vi "YawFromStart.vi"(11 "navX Device":T1 {"Interface"."Update Rate (4Hz-60Hz)" min=4 max=60 step=1}) -> (3 "Yaw":dbl)   [LabVIEW 2015]
uses:
  NavX/navX Library v2/TypeDefs/Z900_navX_DeviceTypeDef.ctl
  NavX/navX Library v2/TypeDefs/Z900_navX_ProtocolTypeDef.ctl
  NavX/navX Library v2/TypeDefs/Z900_navX_NotifyPacketTypeDef.ctl
  NavX/navX Library v2/TypeDefs/Z900_navX_ActionTypeDef.ctl
  Framework/Robot Global Data.vi
  NavX/navX Library v2/navX Library v2.lvlib
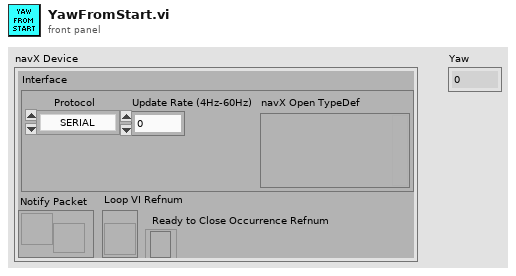
[diagram p1: front panel]
types:
  T1 = typedef "navX Library v2.lvlib/Z900_navX_DeviceTypeDef.ctl" = cluster{"Interface":cluster{"Protocol":T2, "Update Rate (4Hz-60Hz)":u8, "navX Open TypeDef":variant}, "Notify Packet":refnum<notifier>, "Loop VI Refnum":refnum<vi>, "Ready to Close Occurrence Refnum":refnum<k4>}
  T2 = typedef "navX Library v2.lvlib/Z900_navX_ProtocolTypeDef.ctl" = enum16{"SERIAL", "I2C", "SPI"}
  T3 = cluster{"Yaw":dbl, "Roll":dbl, "Pitch":dbl, "Heading":dbl, "Fused Heading":dbl}
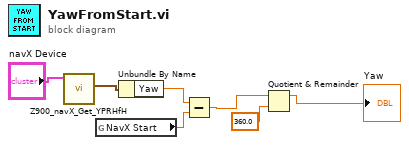
[diagram p0: block diagram]
diagram:
  n1 = call "Z900_navX_Get_YPRHfH.vi"("navX Device"="navX Device") -> ("YRPHfH"=w7:T3)  [unwired: 7 in, 3 out]
  n2 = global read "Robot Global Data.vi" "NavX Start"() -> (w4:dbl)
  n3 = Unbundle By Name(w7) -> ("Yaw"=w5:dbl)
  n4 = Subtract(x=w5, y=w4) -> (x-y=w3:dbl)
  n5 = Quotient & Remainder(x=w3, y=360.0) -> (x-y*floor(x/y)=→"Yaw":dbl)  [unwired: 1 out]
